vi "Meas SMU_MultiChannel.vi"(8 "error in (no error)":errorcluster, 9 "Pins":string[](array[string]), 11 "Semiconductor Module Context":T1) -> (0 "error out":errorcluster, 1 "current measurements":dbl[][](array[numeric]), 2 "voltage measurements":dbl[][](array[numeric]), 3 "Semiconductor Module Context Out":T1)   [LabVIEW 2013]
uses:
  <vilib>/NI_TestStand_SemiconductorModule/NI_TestStand_Semiconductor_Module.lvlibp/PinMap/General/SemiconductorModuleContext.ctl
  <vilib>/NI_TestStand_SemiconductorModule/NI_TestStand_Semiconductor_Module.lvlibp/PinMap/DC Power/PinsToNIDCPowerSessions.vi
  <vilib>/NI_TestStand_SemiconductorModule/NI_TestStand_Semiconductor_Module.lvlibp
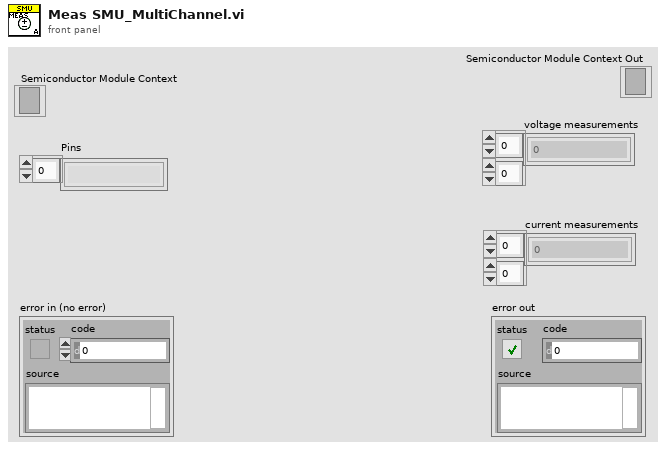
[diagram p1: front panel]
types:
  T1 = typedef "NI_TestStand_Semiconductor_Module.lvlibp/SemiconductorModuleContext.ctl" = refnum<k7>
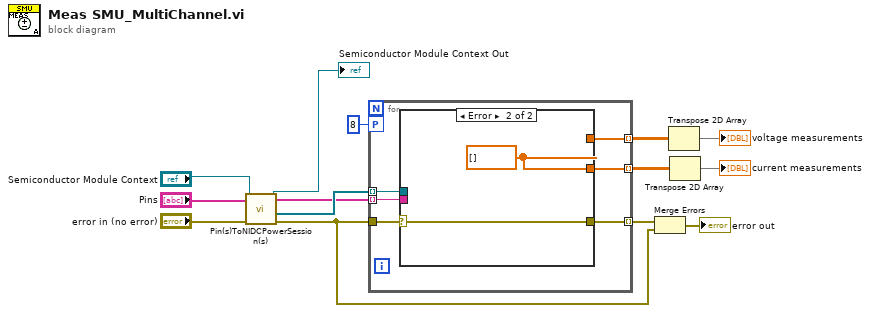
[diagram p0: block diagram]
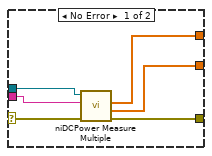
[diagram p2: hidden frame]
diagram:
  n1 = call-poly <vilib>:"Pin(s)ToNIDCPowerSession(s).vi"("error in (no error)"="error in (no error)", "Pins"="Pins", "Semiconductor Module Context"="Semiconductor Module Context") -> ("error out"=w10:errorcluster, "Instrument Sessions"=w14:refnum<k15>[], "Channel Lists"=w13:string[], "Semiconductor Module Context Out"=→"Semiconductor Module Context Out":T1)  [unwired: 4 in, 1 out]
  n2 = for {
    tunnel: w14 -> [w20] mode=indexing
    tunnel: w13 -> [w19] mode=indexing
    tunnel: [w18] -> w5 mode=indexing
    tunnel: w10 -> [w17]
    tunnel: [w16] -> w7 mode=indexing
    tunnel: [w15] -> w11 mode=indexing
    workers-P: 8 -> [_]
    n3 = case shown="Error" w17 {
      selector: w17 -> [w22 w28]
      tunnel: [w24 w28] -> w15
      tunnel: w20 -> [w21 _]
      tunnel: w19 -> [w23 _]
      tunnel: [w26 w27] -> w16
      tunnel: [w25 w27] -> w18
      frame No Error {
        n4 = call <instrlib>:"niDCPower Measure Multiple.vi"("error in (no error)"=w22, "channel name"=w23, "instrument handle"=w21) -> ("error out"=w24:errorcluster, "current measurements"=w25:dbl[], "voltage measurements"=w26:dbl[])  [unwired: 5 in, 1 out]
      }
      frame Error {
        w27 = dbl[] [] ("voltage measurements")
      }
    }
  }
  n5 = Merge Errors(w11, w10) -> (→"error out":errorcluster)
  n6 = Transpose 2D Array(2D array=w7) -> (transposed array=→"voltage measurements":dbl[][])
  n7 = Transpose 2D Array(2D array=w5) -> (transposed array=→"current measurements":dbl[][])
